vi "IDToStr.vi"(1 "帧ID输入":u32 max=4096 step=1) -> (0 "帧ID输出":string)   [LabVIEW 2013]
panel:
  out "error out":errorcluster caption="错误输出"
  in  "error in":errorcluster caption="错误输入"
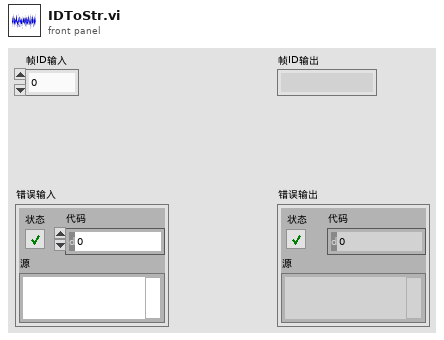
[diagram p1: front panel]
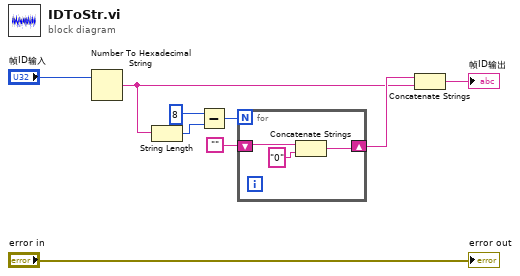
[diagram p0: block diagram]
diagram:
  n1 = Number To Hexadecimal String(2:"帧ID输入") -> (0:w3:string)  [unwired: 1 in]
  n2 = String Length(string=w3) -> (length=w7:i32)
  n3 = Subtract(x=8, y=w7) -> (x-y=w6:i32)
  n4 = for {
    N: w6 -> [_]
    shift-right: [w11] -> w4
    shift-left: "" -> [w12]
    n5 = Concatenate Strings(w12, "0") -> (w11:string)
  }
  n6 = Concatenate Strings(w4, w3) -> (→"帧ID输出":string)
  "error out" <- "error in"
